vi "GB_INV B Current Sense.vi"(8 "error in (no error)":errorcluster, 11 "ControlBoard VISA":refnum<visa-resource-name>="ControlBoard") -> (0 "error out":errorcluster, 3 "Current Readings":dbl[](array[numeric]))   [LabVIEW 2022 SP3]
uses:
  Serial Board Com/ADCSelector GB.ctl
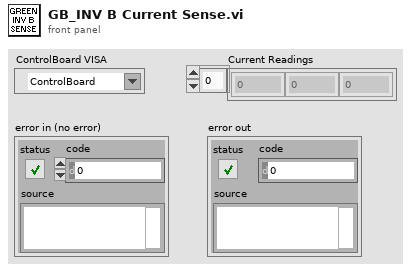
[diagram p1: front panel]
types:
  T1 = typedef "ADCSelector GB.ctl" = enum16{"INVA_ISENSE_U", "INVA_ISENSE_V", "INVA_ISENSE_W", "INVA_UDC", "INVA_TEMP", "HB_ISENSE", "AUX_ISENSE_U", "AUX_ISENSE_V", "AUX_ISENSE_W", "VLINE_AB", "VLINE_BC", "VLINE_CA", "REF_1P5V", "VSENSE_POS_24V", "VSENSE_POS_5V", "VSENSE_NEG_15V", "TEST_POINT", "INVB_ISENSE_U", "INVB_ISENSE_V", "INVB_ISENSE_W", "INVB_UDC", "INVB_TEMP", "HB_TEMP", "AUXA_TEMP", "AUXB_TEMP", "AUXC_TEMP", "VOUT_AB", "VOUT_BC", "VOUT_CA", "REF_2P5V", "VSENSE_POS_15V", "VSENSE_POS_3P3V", "NET_ANALYZER"}
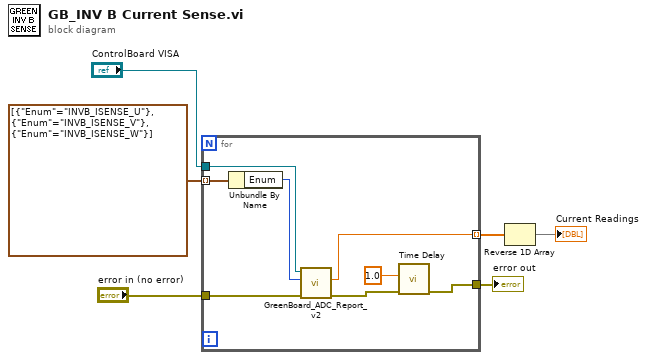
[diagram p0: block diagram]
diagram:
  n1 = for {
    tunnel: cluster{"Enum":T1}[] [{"Enum"=enum."INVB_ISENSE_U"}, {"Enum"=enum."INVB_ISENSE_V"}, {"Enum"=enum."INVB_ISENSE_W"}] -> [w12] mode=indexing
    tunnel: [w14] -> w6 mode=indexing
    tunnel: [w10] -> w1
    tunnel: "error in (no error)" -> [w13]
    tunnel: "ControlBoard VISA" -> [w7]
    n2 = Unbundle By Name(w12) -> ("Enum"=w9:T1)
    n3 = call "GreenBoard_ADC_Report_v2.vi"("error in (no error)"=w13, "Green Board Enum"=w9, "ControlBoard VISA"=w7) -> ("error out"=w11:errorcluster, "Result"=w14:dbl)  [unwired: 5 in, 2 out]
    n4 = call "Time Delay"("error in (no error)"=w11, "Delay Time (s)"=1.0) -> ("error out"=w10:errorcluster)  [unwired: 9 in]
  }
  "error out" <- w1
  n5 = Reverse 1D Array(array=w6) -> (reversed array=→"Current Readings":dbl[])
